vi "svfa_Build Spectrum Info (Dual).vi"(0 "scaled signal  X [EU]":waveform(dbl)={"t0"=timestamp(0 s since 1904-01-01), "dt"=0.0, "Y"=[]}, 1 "processing control":T7(ring), 5 "scaled signal  Y [EU]":waveform(dbl)={"t0"=timestamp(0 s since 1904-01-01), "dt"=0.0, "Y"=[]}, 7 "window":T8 items=["None"=0, "Hanning"=1, "Hamming"=2, "Blackman-Harris"=3, "Exact Blackman"=4, "Blackman"=5, "Flat Top"=6, "4 Term B-Harris "=7, "7 Term B-Harris"=8, "Low Sidelobe"=9, "Force - Exponential"=10, "Blackman Nuttall"=11, "Triangle"=30, "Bartlett-Hanning"=31, "Bohman"=32, "Parzen"=33, "Welch"=34, "Kaiser"=60, "Dolph-Chebyshev"=61, "Gaussian"=62], 8 "x-channel index":i32, 9 "window size":i32, 10 "y-channel index":i32, 11 "error in (no error)":errorcluster, 12 "spectrum type":T3, 13 "spectrum info in":T1={"channel name"="", "description"="", "x-axis units"=0, "spectral info"={"spectrum type"=enum."Power [Magnitude^2]", "linear/dB"=enum."linear", "window"=0, "window size"=0, "FFT size"=0}, "engineering units"=0, "custom label"="", "dB reference [EU]"=0.0, "peak units"=enum."rms", "weighting filter"=0, "spectral density?"=FALSE, "unit label"="", "spectrum skewed?"=FALSE, "complimentary spectrum units"=enum."none"} {"x-axis units" items=["Time (s)"=0, "Frequency-CB (Hz)"=1, "Frequency-CPB (Hz)"=1248, "Frequency-Arbitrary (Hz)"=2357, "Quefrency (s)"=2, "Revolutions (rev)"=3, "Order"=4, "Speed (RPM)"=11, "Speed (rad/s)"=21, "Index"=65535]; "weighting filter" items=["Linear", "A-weighting", "B-weighting", "C-weighting", "ITU-R 468-4", "Dolby", "CCITT", "C-message", "Wb", "Wc", "Wd", "We", "Wf", "Wh", "Wj", "Wk", "Wm", "AES17 20 kHz lowpass", "AES17 40 kHz lowpass", "AES17 20 kHz highpass", "AES17 40 kHz highpass"]; "dB reference [EU]" format="%.2f"; "engineering units" items=["custom..."=0, "V"=1, "A"=21, "C"=30, "pC"=31, "s"=32, "-"=29, "Pa"=2, "N"=20, "g"=3, "m/s^2"=4, "m/s"=5, "m"=6, "mm/s"=12, "mm"=13, "micron/s"=14, "micron"=15, "in/s^2"=7, "in/s"=8, "in"=9, "mil/s"=10, "mil"=11, "rad/s^2"=16, "rad/s"=17, "rad"=18, "deg/s^2"=26, "deg/s"=27, "deg"=28, "RPM"=22, "cycle/s^2"=23, "Hz"=24, "cycle"=25, "strain"=19]; "spectral info"."window" items=["None "=0, "Hanning"=1, "Hamming"=2, "Blackman-Harris"=3, "Exact Blackman"=4, "Blackman"=5, "Flat Top"=6, "4 Term B-Harris "=7, "7 Term B-Harris"=8, "Low Sidelobe"=9, "Force - Exponential"=10, "Gaussian"=62]}, 14 "x-axis units":u16(ring)=1 items=["time"=0, "frequency"=1, "quefrency"=2, "revolutions"=3, "order"=4, "rpm"=11]) -> (2 "spectrum info out":T1={"channel name"="", "description"="", "x-axis units"=0, "spectral info"={"spectrum type"=enum."Power [Magnitude^2]", "linear/dB"=enum."linear", "window"=0, "window size"=0, "FFT size"=0}, "engineering units"=0, "custom label"="", "dB reference [EU]"=0.0, "peak units"=enum."rms", "weighting filter"=0, "spectral density?"=FALSE, "unit label"="", "spectrum skewed?"=FALSE, "complimentary spectrum units"=enum."none"} {"x-axis units" items=["Time (s)"=0, "Frequency-CB (Hz)"=1, "Frequency-CPB (Hz)"=1248, "Frequency-Arbitrary (Hz)"=2357, "Quefrency (s)"=2, "Revolutions (rev)"=3, "Order"=4, "Speed (RPM)"=11, "Speed (rad/s)"=21, "Index"=65535]; "weighting filter" items=["Linear", "A-weighting", "B-weighting", "C-weighting", "ITU-R 468-4", "Dolby", "CCITT", "C-message", "Wb", "Wc", "Wd", "We", "Wf", "Wh", "Wj", "Wk", "Wm", "AES17 20 kHz lowpass", "AES17 40 kHz lowpass", "AES17 20 kHz highpass", "AES17 40 kHz highpass"]; "dB reference [EU]" format="%.2f"; "engineering units" items=["custom..."=0, "V"=1, "A"=21, "C"=30, "pC"=31, "s"=32, "-"=29, "Pa"=2, "N"=20, "g"=3, "m/s^2"=4, "m/s"=5, "m"=6, "mm/s"=12, "mm"=13, "micron/s"=14, "micron"=15, "in/s^2"=7, "in/s"=8, "in"=9, "mil/s"=10, "mil"=11, "rad/s^2"=16, "rad/s"=17, "rad"=18, "deg/s^2"=26, "deg/s"=27, "deg"=28, "RPM"=22, "cycle/s^2"=23, "Hz"=24, "cycle"=25, "strain"=19]; "spectral info"."window" items=["None "=0, "Hanning"=1, "Hamming"=2, "Blackman-Harris"=3, "Exact Blackman"=4, "Blackman"=5, "Flat Top"=6, "4 Term B-Harris "=7, "7 Term B-Harris"=8, "Low Sidelobe"=9, "Force - Exponential"=10, "Gaussian"=62]}, 3 "dup processing control":T7(ring), 4 "dup scaled signal  X [EU]":waveform(dbl), 6 "dup scaled signal  Y [EU]":waveform(dbl), 15 "error out":errorcluster)   [LabVIEW 2017]
uses:
  <vilib>/addons/_NISVFA/_Shared subVIs/Controls/svc_Spectrum Info.ctl
  <vilib>/addons/_NISVFA/_Shared subVIs/Controls/svc_X-Axis Units.ctl
  <vilib>/addons/_NISVFA/_Shared subVIs/Controls/svc_Spectrum Type.ctl
  <vilib>/addons/_NISVFA/_Shared subVIs/Controls/svc_Engineering Units Text Ring.ctl
  <vilib>/addons/_NISVFA/_Shared subVIs/Controls/svc_Weighting Filter Text Ring.ctl
  <vilib>/addons/_NISVFA/_Shared subVIs/Controls/svc_Complimentary Spectrum Units.ctl
  <vilib>/addons/_NISVFA/_Shared subVIs/Controls/svc_Window [Dual FFT].ctl
  <vilib>/addons/_NISVFA/_Shared subVIs/Common/svc_Engineering Units to Unit Label.vi
  <vilib>/addons/_NISVFA/_Shared subVIs/Common/svc_Unit Label to Engineering Units.vi
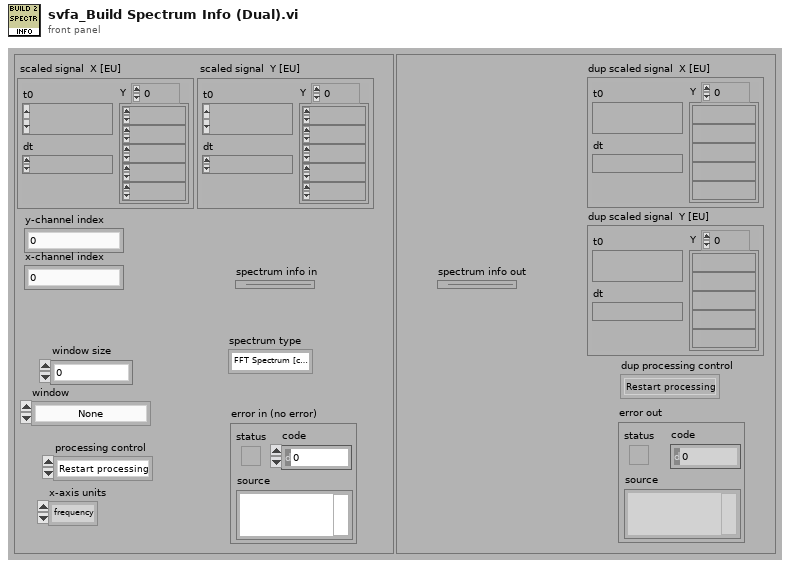
[diagram p1: front panel]
types:
  T1 = typedef "svc_Spectrum Info.ctl" = cluster{"channel name":string, "description":string, "x-axis units":T2, "spectral info":cluster{"spectrum type":T3, "linear/dB":enum16{"linear", "dB"}, "window":u16, "window size":i32, "FFT size":i32}, "engineering units":T4, "custom label":string, "dB reference [EU]":dbl, "peak units":enum16{"rms", "peak", "peak-peak"}, "weighting filter":T5, "spectral density?":bool, "unit label":string, "spectrum skewed?":bool, "complimentary spectrum units":T6}
  T2 = typedef "svc_X-Axis Units.ctl" = u16
  T3 = typedef "svc_Spectrum Type.ctl" = enum16{"FFT Spectrum [complex]", "Amplitude [Magnitude]", "Power [Magnitude^2]", "Cross Spectrum [complex]", "Frequency Response [Complex]"}
  T4 = typedef "svc_Engineering Units Text Ring.ctl" = u16
  T5 = typedef "svc_Weighting Filter Text Ring.ctl" = u16
  T6 = typedef "svc_Complimentary Spectrum Units.ctl" = enum16{"none", "radians", "degrees", "cycles", "imaginary"}
  T7 = enum16{"Restart processing", "Continue processing", "Skip processing"}
  T8 = typedef "svc_Window [Dual FFT].ctl" = u32
  T9 = typedef "svc_Channel Info.ctl" = cluster{"sensor sensitivity":dbl, "engineering units":T4, "dB reference":dbl, "custom label":string, "weighting filter":T5, "pregain":dbl}
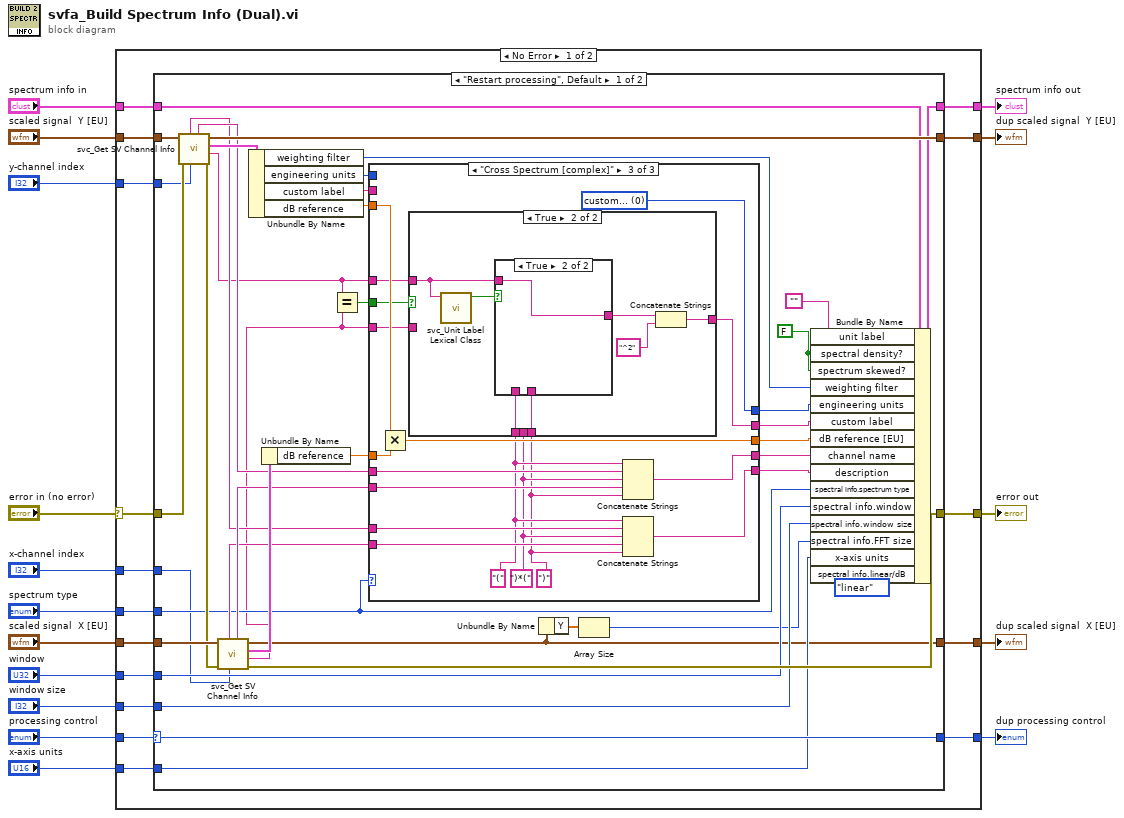
[diagram p0: block diagram]
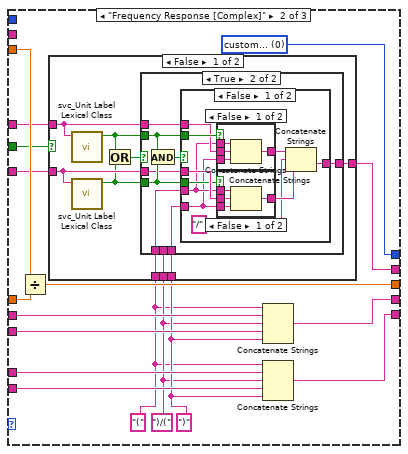
[diagram p3: hidden frame]
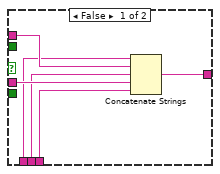
[diagram p4: hidden frame]
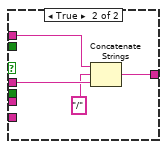
[diagram p7: hidden frame]
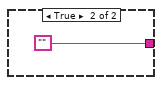
[diagram p8: hidden frame]
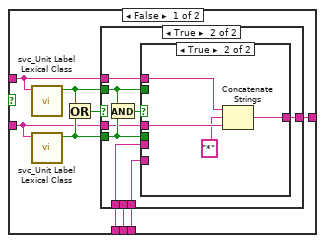
[diagram p9: hidden frame]
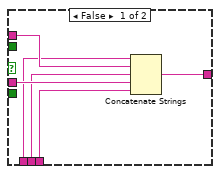
[diagram p10: hidden frame]
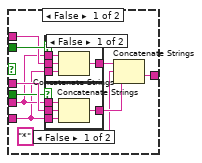
[diagram p11: hidden frame]
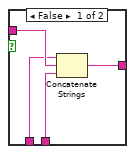
[diagram p14: hidden frame]
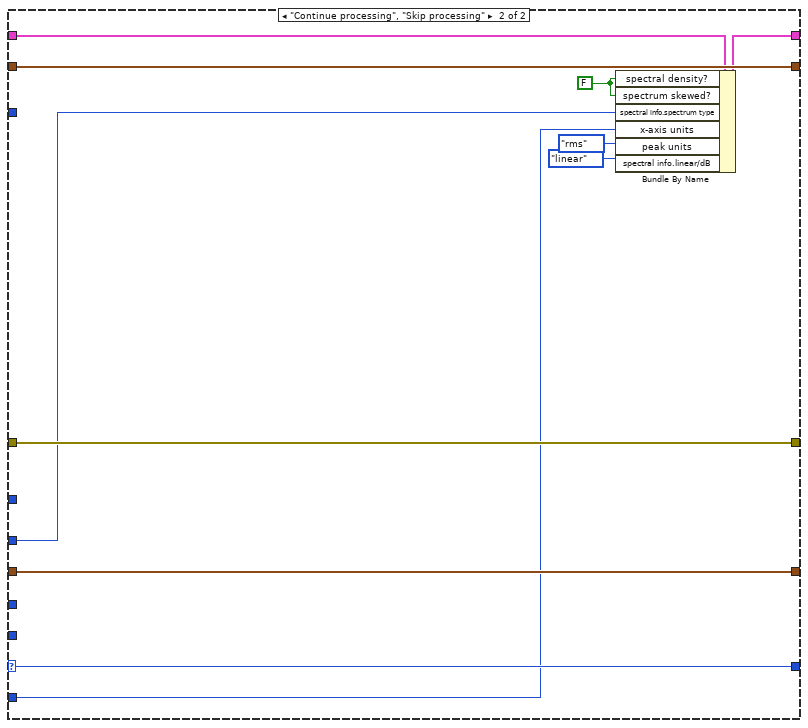
[diagram p15: hidden frame]
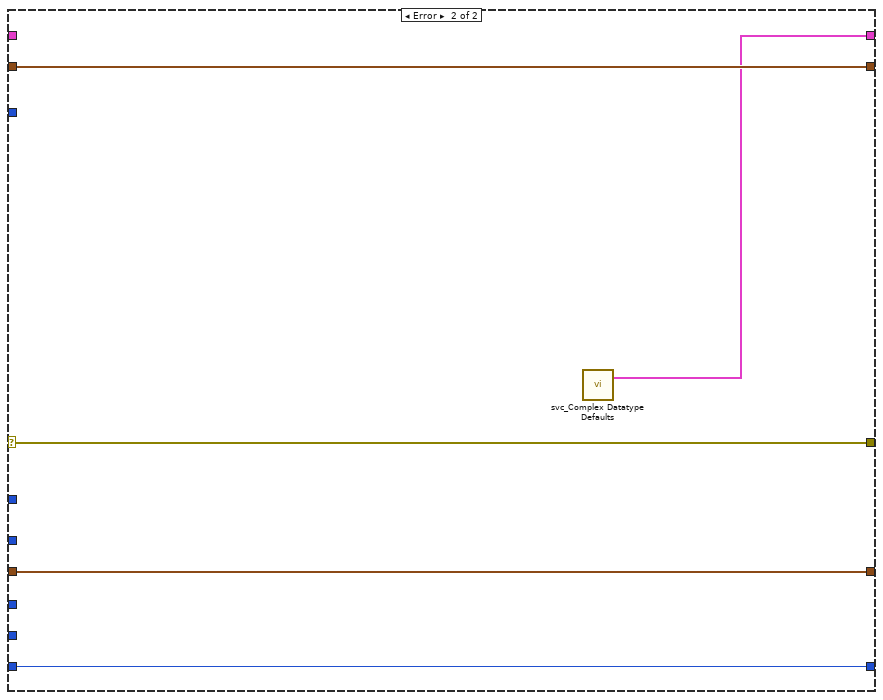
[diagram p16: hidden frame]
diagram:
  n1 = case shown="No Error" "error in (no error)" {
    selector: "error in (no error)" -> [w27 w234]
    tunnel: [w23 w231] -> w16
    tunnel: "scaled signal  X [EU]" -> [w32 w233]
    tunnel: [w31 w233] -> w8
    tunnel: [w26 w234] -> w14
    tunnel: "scaled signal  Y [EU]" -> [w30 w232]
    tunnel: [w29 w232] -> w7
    tunnel: "spectrum type" -> [w28 _]
    tunnel: "window" -> [w25 _]
    tunnel: "window size" -> [w24 _]
    tunnel: "processing control" -> [w22 w230]
    tunnel: [w21 w230] -> w6
    tunnel: "x-axis units" -> [w20 _]
    tunnel: "spectrum info in" -> [w19 _]
    tunnel: "x-channel index" -> [w18 _]
    tunnel: "y-channel index" -> [w17 _]
    frame No Error {
      n2 = case shown="\"Restart processing\", Default" w22 {
        selector: w22 -> [w55 w226]
        tunnel: [w42 w221] -> w23
        tunnel: w32 -> [w72 w227]
        tunnel: [w36 w227] -> w31
        tunnel: w30 -> [w70 w229]
        tunnel: [w68 w229] -> w29
        tunnel: w28 -> [w40 w219]
        tunnel: w27 -> [w64 w228]
        tunnel: [w62 w228] -> w26
        tunnel: w25 -> [w56 _]
        tunnel: w24 -> [w48 _]
        tunnel: w19 -> [w43 w222]
        tunnel: [w55 w226] -> w21
        tunnel: w20 -> [w44 w224]
        tunnel: w18 -> [w34 _]
        tunnel: w17 -> [w33 _]
        frame "Restart processing", Default {
          w52 = FALSE ("spectrum skewed?")
          n3 = call <vilib>:"svc_Get SV Channel Info.vi"("channel index"=w33, "error in (no error)"=w64, "scaled signal [EU]"=w70) -> ("error out"=w63:errorcluster, "unit label"=w39:string, "channel info"=w69:T9, "dup scaled signal [EU]"=w68:waveform(dbl), "channel name"=w50:string, "channel description"=w46:string)  [unwired: 3 in]
          n4 = call <vilib>:"svc_Get SV Channel Info.vi"("channel index"=w34, "error in (no error)"=w63, "scaled signal [EU]"=w72) -> ("error out"=w62:errorcluster, "unit label"=w38:string, "channel info"=w71:T9, "dup scaled signal [EU]"=w36:waveform(dbl), "channel name"=w51:string, "channel description"=w47:string)  [unwired: 3 in]
          n5 = Unbundle By Name(w69) -> ("weighting filter"=w61:T5, "engineering units"=w58:T4, "custom label"=w59:string, "dB reference"=w60:dbl)
          n6 = Unbundle By Name(w71) -> ("dB reference"=w67:dbl)
          n7 = Equal?(x=w39, y=w38) -> (x = y?=w65:bool)
          n8 = case shown="\"Cross Spectrum [complex]\"" w40 {
            tunnel: w60 -> [w74 w94 w159]
            tunnel: w67 -> [_ w93 w158]
            tunnel: [w74 w92 w157] -> w66
            tunnel: w65 -> [_ w91 w144]
            tunnel: w39 -> [_ w90 w143]
            tunnel: [w77 w89 w149] -> w57
            tunnel: w38 -> [_ w88 w145]
            tunnel: [w76 w87 w156] -> w54
            tunnel: w59 -> [w77 _ _]
            tunnel: w58 -> [w76 _ _]
            tunnel: w51 -> [_ w85 w155]
            tunnel: w50 -> [w75 w86 w154]
            tunnel: [w75 w84 w153] -> w49
            tunnel: w47 -> [_ w82 w152]
            tunnel: w46 -> [w73 w83 w151]
            tunnel: [w73 w78 w150] -> w45
            frame "Power [Magnitude^2]", Default {
            }
            frame "Frequency Response [Complex]" {
              w80 = ")/(" ("Substring")
              w81 = ")" ("Substring")
              w79 = "(" ("Substring")
              w87 = T4 0 items=["custom..."=0, "V"=1, "A"=21, "Pa"=2, "N"=20, "g"=3, "m/s^2"=4, "m/s"=5, "m"=6, "mm/s"=12, "mm"=13, "microns/s"=14, "microns"=15, "in/s^2"=7, "in/s"=8, "in"=9, "mils/s"=10, "mils"=11, "rad/s^2"=16, "rad/s"=17, "rad"=18, "strain"=19] ("engineering units")
              n9 = Divide(x=w94, y=w93) -> (x/y=w92:dbl)
              n10 = case shown="False" w91 {
                tunnel: w90 -> [w99 _]
                tunnel: [w103 "" ("Empty String Constant")] -> w89
                tunnel: w88 -> [w98 _]
                tunnel: w81 -> [w102 _]
                tunnel: w80 -> [w101 _]
                tunnel: w79 -> [w100 _]
                frame False {
                  n11 = call <vilib>:"svc_Unit Label Lexical Class.vi"("unit label"=w99) -> ("letters only?"=w96:bool)  [unwired: 6 in]
                  n12 = call <vilib>:"svc_Unit Label Lexical Class.vi"("unit label"=w98) -> ("letters only?"=w95:bool)  [unwired: 6 in]
                  n13 = Or(x=w96, y=w95) -> (x .or. y?=w97:bool)
                  n14 = case shown="True" w97 {
                    tunnel: w99 -> [w109 w114]
                    tunnel: w98 -> [w108 w113]
                    tunnel: [w107 w112] -> w103
                    tunnel: w102 -> [w106 w110]
                    tunnel: w101 -> [w105 _]
                    tunnel: w100 -> [w104 w111]
                    tunnel: w96 -> [_ w116]
                    tunnel: w95 -> [_ w117]
                    frame False {
                      n15 = Concatenate Strings(w104, w109, w105, w108, w106) -> (w107:string)
                    }
                    frame True {
                      n16 = And(x=w116, y=w117) -> (x .and. y?=w115:bool)
                      n17 = case shown="False" w115 {
                        tunnel: w117 -> [w124 _]
                        tunnel: w116 -> [w127 _]
                        tunnel: w114 -> [w126 w141]
                        tunnel: w113 -> [w125 w140]
                        tunnel: [w119 w139] -> w112
                        tunnel: w111 -> [w123 _]
                        tunnel: w110 -> [w122 _]
                        frame False {
                          n18 = case shown="False" w127 {
                            tunnel: w126 -> [w136 w137]
                            tunnel: [w133 w137] -> w121
                            tunnel: w123 -> [w135 _]
                            tunnel: w122 -> [w134 _]
                            frame False {
                              n19 = Concatenate Strings(w135, w136, w134) -> (w133:string)
                            }
                            frame True {
                            }
                          }
                          n20 = case shown="False" w124 {
                            tunnel: w125 -> [w131 w132]
                            tunnel: [w130 w132] -> w120
                            tunnel: w123 -> [w129 _]
                            tunnel: w122 -> [w128 _]
                            frame False {
                              n21 = Concatenate Strings(w129, w131, w128) -> (w130:string)
                            }
                            frame True {
                            }
                          }
                          n22 = Concatenate Strings(w121, "/" ("Substring"), w120) -> (w119:string)
                        }
                        frame True {
                          n23 = Concatenate Strings(w141, "/" ("string"), w140) -> (w139:string)
                        }
                      }
                    }
                  }
                }
                frame True {
                }
              }
              n24 = Concatenate Strings(w79, w86, w80, w85, w81) -> (w84:string)
              n25 = Concatenate Strings(w79, w83, w80, w82, w81) -> (w78:string)
            }
            frame "Cross Spectrum [complex]" {
              w147 = ")*(" ("Substring")
              w146 = ")" ("Substring")
              w148 = "(" ("Substring")
              w156 = T4 0 items=["custom..."=0, "V"=1, "A"=21, "Pa"=2, "N"=20, "g"=3, "m/s^2"=4, "m/s"=5, "m"=6, "mm/s"=12, "mm"=13, "microns/s"=14, "microns"=15, "in/s^2"=7, "in/s"=8, "in"=9, "mils/s"=10, "mils"=11, "rad/s^2"=16, "rad/s"=17, "rad"=18, "strain"=19] ("engineering units")
              n26 = Multiply(x=w159, y=w158) -> (x*y=w157:dbl)
              n27 = case shown="True" w144 {
                tunnel: w143 -> [w161 w210]
                tunnel: [w168 w209] -> w149
                tunnel: w145 -> [w160 _]
                tunnel: w146 -> [w167 w207]
                tunnel: w147 -> [w166 _]
                tunnel: w148 -> [w165 w208]
                frame False {
                  n28 = call <vilib>:"svc_Unit Label Lexical Class.vi"("unit label"=w161) -> ("letters only?"=w163:bool)  [unwired: 6 in]
                  n29 = call <vilib>:"svc_Unit Label Lexical Class.vi"("unit label"=w160) -> ("letters only?"=w162:bool)  [unwired: 6 in]
                  n30 = Or(x=w163, y=w162) -> (x .or. y?=w164:bool)
                  n31 = case shown="True" w164 {
                    tunnel: w161 -> [w174 w179]
                    tunnel: w160 -> [w173 w178]
                    tunnel: [w172 w177] -> w168
                    tunnel: w167 -> [w171 w175]
                    tunnel: w166 -> [w170 _]
                    tunnel: w165 -> [w169 w176]
                    tunnel: w163 -> [_ w181]
                    tunnel: w162 -> [_ w182]
                    frame False {
                      n32 = Concatenate Strings(w169, w174, w170, w173, w171) -> (w172:string)
                    }
                    frame True {
                      n33 = And(x=w181, y=w182) -> (x .and. y?=w180:bool)
                      n34 = case shown="True" w180 {
                        tunnel: w182 -> [w189 _]
                        tunnel: w181 -> [w192 _]
                        tunnel: w179 -> [w191 w206]
                        tunnel: w178 -> [w190 w205]
                        tunnel: [w184 w204] -> w177
                        tunnel: w176 -> [w188 _]
                        tunnel: w175 -> [w187 _]
                        frame False {
                          n35 = case shown="False" w192 {
                            tunnel: w191 -> [w201 w202]
                            tunnel: [w198 w202] -> w186
                            tunnel: w188 -> [w200 _]
                            tunnel: w187 -> [w199 _]
                            frame False {
                              n36 = Concatenate Strings(w200, w201, w199) -> (w198:string)
                            }
                            frame True {
                            }
                          }
                          n37 = case shown="False" w189 {
                            tunnel: w190 -> [w196 w197]
                            tunnel: [w195 w197] -> w185
                            tunnel: w188 -> [w194 _]
                            tunnel: w187 -> [w193 _]
                            frame False {
                              n38 = Concatenate Strings(w194, w196, w193) -> (w195:string)
                            }
                            frame True {
                            }
                          }
                          n39 = Concatenate Strings(w186, "*" ("Substring"), w185) -> (w184:string)
                        }
                        frame True {
                          n40 = Concatenate Strings(w206, "*" ("string"), w205) -> (w204:string)
                        }
                      }
                    }
                  }
                }
                frame True {
                  n41 = call <vilib>:"svc_Unit Label Lexical Class.vi"("unit label"=w210) -> ("letters only?"=w213:bool)  [unwired: 6 in]
                  n42 = case shown="True" w213 {
                    tunnel: [w216 w218] -> w211
                    tunnel: w210 -> [w217 w218]
                    tunnel: w208 -> [w215 _]
                    tunnel: w207 -> [w214 _]
                    frame False {
                      n43 = Concatenate Strings(w215, w217, w214) -> (w216:string)
                    }
                    frame True {
                    }
                  }
                  n44 = Concatenate Strings(w211, "^2" ("Substring")) -> (w209:string)
                }
              }
              n45 = Concatenate Strings(w148, w154, w147, w155, w146) -> (w153:string)
              n46 = Concatenate Strings(w148, w151, w147, w152, w146) -> (w150:string)
            }
          }
          n47 = Unbundle By Name(w36) -> ("Y"=w37:dbl[])
          n48 = Array Size(array=w37) -> (size(s)=w35:i32)
          n49 = Bundle By Name(cluster=w43, "unit label"="" ("Empty String Constant"), "spectral density?"=w52, "spectrum skewed?"=w52, "weighting filter"=w61, "engineering units"=w54, "custom label"=w57, "dB reference [EU]"=w66, "channel name"=w49, "description"=w45, "spectral info.spectrum type"=w40, "spectral info.window"=w56, "spectral info.window size"=w48, "spectral info.FFT size"=w35, "x-axis units"=w44, "spectral info.linear/dB"=enum16{"linear", "dB"}."linear") -> (w42:T1)
        }
        frame "Continue processing", "Skip processing" {
          w223 = FALSE ("spectral density?")
          n50 = Bundle By Name(cluster=w222, "spectral density?"=w223, "spectrum skewed?"=w223, "spectral info.spectrum type"=w219, "x-axis units"=w224, "peak units"=enum16{"rms", "peak", "peak-peak"}."rms", "spectral info.linear/dB"=enum16{"linear", "dB"}."linear") -> (w221:T1)
        }
      }
    }
    frame Error {
      n51 = call <vilib>:"svc_Complex Datatype Defaults.vi"() -> ("dead spectrum info"=w231:T1)  [unwired: 11 in, 8 out]
    }
  }
  "spectrum info out" <- w16
  "error out" <- w14
  "dup processing control" <- w6
  "dup scaled signal  X [EU]" <- w8
  "dup scaled signal  Y [EU]" <- w7
